vi "Write SPI_FRM_Array.vi"(8 "error in (no error)":errorcluster, 10 "SPI_FRM_Array":T1[](array[typedef]) {"Addr" format="%x"; "Data" format="%x"}, 11 "Config_Read_SPI in":refnum<class "Config_Read_SPI.lvclass">) -> (0 "error out":errorcluster, 3 "Config_Read_SPI out":refnum<class "Config_Read_SPI.lvclass">)   [LabVIEW 2018, in "Config_Read_SPI.lvclass"]
uses:
  Config_Read_SPI.lvclass
  SPI_FRM_Config.ctl
  Classes/Config_Read/RW_Option.ctl
  SPI_Mode.ctl
  Config_Read_SPI.lvclass/Config_Read_SPI.ctl
  Classes/Config_Read/Config_Read_BML.lvclass
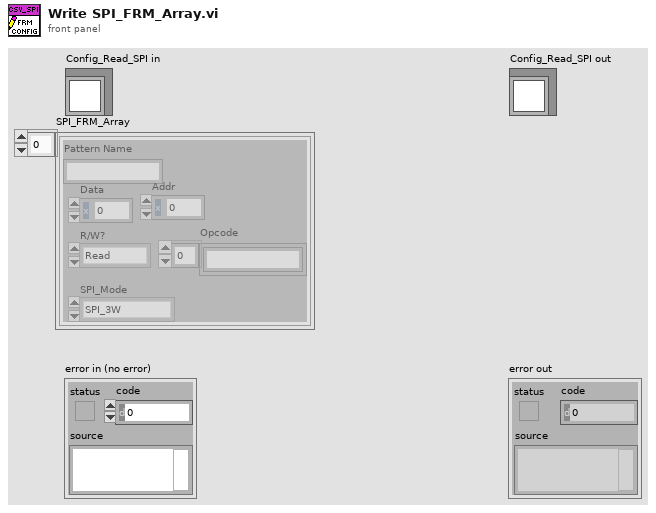
[diagram p1: front panel]
types:
  T1 = typedef "Config_Read_SPI.lvclass/SPI_FRM_Config.ctl" = cluster{"Pattern Name":string, "Data":u16, "Addr":u16, "R/W?":T2, "Opcode":string[], "SPI_Mode":T3}
  T2 = typedef "Config_Read_BML.lvclass/RW_Option.ctl" = enum16{"Read", "Write", "R/W"}
  T3 = typedef "Config_Read_SPI.lvclass/SPI_Mode.ctl" = enum16{"SPI_3W", "SPI_4W"}
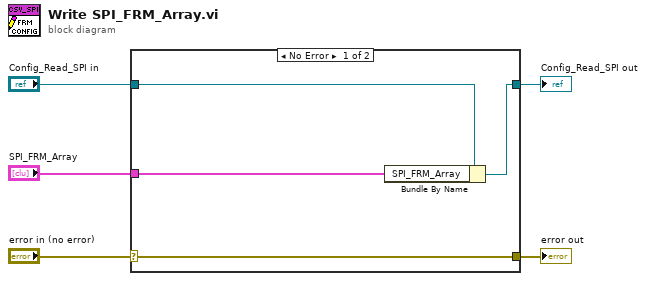
[diagram p0: block diagram]
diagram:
  n1 = case shown="No Error" "error in (no error)" {
    selector: "error in (no error)" -> [w9 w10]
    tunnel: [w9 w10] -> w4
    tunnel: [w7 w11] -> w2
    tunnel: "Config_Read_SPI in" -> [w8 w11]
    tunnel: "SPI_FRM_Array" -> [w6 _]
    frame No Error {
      n2 = Bundle By Name(cluster=w8, "SPI_FRM_Array"=w6) -> (w7:refnum<class "Config_Read_SPI.lvclass">)
    }
    frame Error {
    }
  }
  "error out" <- w4
  "Config_Read_SPI out" <- w2
